vi "Create XRay Cabinet.vi"(8 "error in (no error)":errorcluster, 11 "3D Picture":refnum<vi>) -> (0 "error out":errorcluster, 3 "XRay Cabinet out":refnum<class "XRay Cabinet.lvclass">)   [LabVIEW 2026, in "XRay Cabinet.lvclass"]
uses:
  XRay Cabinet.lvclass
  XRay Scene/XRay Scene.lvclass
  XRay Cabinet.lvclass/XRay Cabinet.ctl
  <vilib>/picture/3D Picture Control/Object/Create Object (name).vi
  <vilib>/picture/3D Picture Control/Object/Add Object (no reference).vi
  <vilib>/picture/3D Picture Control/NI_3D Picture Control.lvlib
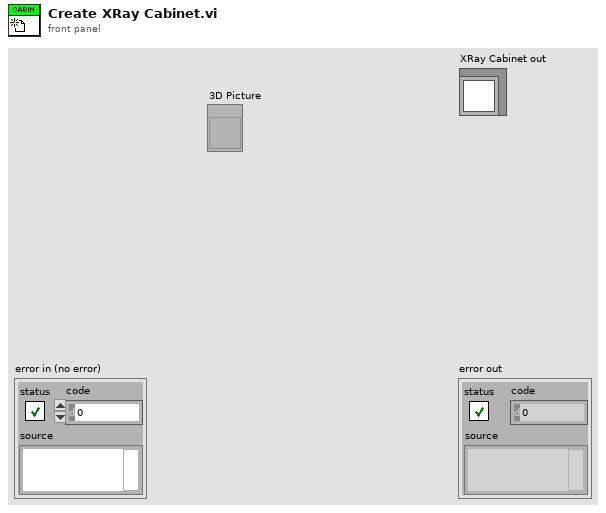
[diagram p1: front panel]
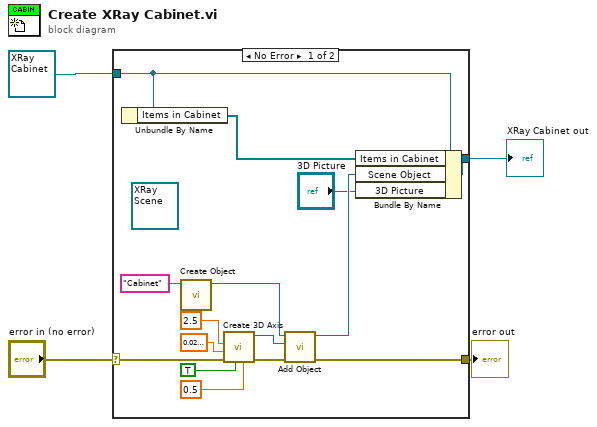
[diagram p0: block diagram]
diagram:
  n1 = case shown="No Error" "error in (no error)" {
    selector: "error in (no error)" -> [w10 w20]
    tunnel: [w9 w20] -> w3
    tunnel: [w19 w21] -> w1
    tunnel: refnum<class "XRay Cabinet.lvclass"> refnum ("XRay Cabinet in") -> [w8 w21]
    frame No Error {
      (unwired) refnum<class "XRay Scene.lvclass"> refnum ("XRay Scene.lvclass")
      n2 = Unbundle By Name(w8) -> ("Items in Cabinet"=w7:refnum<class "XRay Scene.lvclass">[])
      n3 = call-poly <vilib>:"Create Object.vi"("Name"="Cabinet") -> ("Scene:New Object"=w12:refnum<vi>)  [unwired: 9 in, 1 out]
      n4 = call <vilib>:"Create 3D Axis.vi"("Character Size"=sgl 0.5, "Axis label?"=TRUE, "error in (no error)"=w10, "Radius"=sgl 0.03, "Length"=sgl 2.5 ("Height")) -> ("error out"=w13:errorcluster, "New Object Refnum"=w14:refnum<vi>)  [unwired: 5 in]
      n5 = call-poly <vilib>:"Add Object.vi"("error in (no error)"=w13, "New Object In"=w14, "Scene Object In"=w12) -> ("error out"=w9:errorcluster, "Scene Object Out"=w6:refnum<vi>)  [unwired: 7 in]
      n6 = Bundle By Name(cluster=w8, "Items in Cabinet"=w7, "Scene Object"=w6, "3D Picture"="3D Picture") -> (w19:refnum<class "XRay Cabinet.lvclass">)
    }
    frame Error {
    }
  }
  "error out" <- w3
  "XRay Cabinet out" <- w1
